vi "MTM2_getSample_tangentActuatorSteps.vi"(8 "error in (no error)":errorcluster, 11 "tangentActuatorSteps_Ctl":T1={"private_rcvStamp"=0.0, "steps[6]"=[0, 0, 0, 0, 0, 0]}) -> (0 "error out":errorcluster, 2 "function return":i32, 3 "tangentActuatorSteps_Ctl out":T1)   [LabVIEW 2018, in "SALLV_MTM2.lvlib"]
doc: "int MTM2_shm_getSample_tangentActuatorStepsLV(MTM2_tangentActuatorStepsLV *tangentActuatorSteps_Ctl );"
uses:
  DataTypes/tangentActuatorSteps.ctl
  SALLV_MTM2.lvlib
  SALLV_MTM2.so
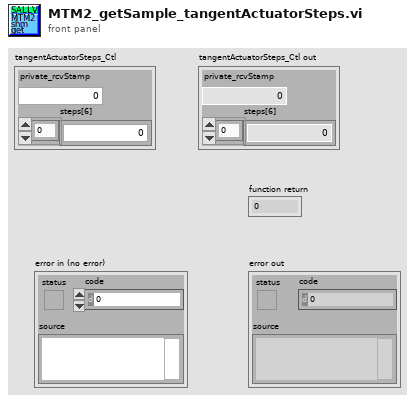
[diagram p1: front panel]
types:
  T1 = typedef "SALLV_MTM2.lvlib/tangentActuatorSteps.ctl" = cluster{"private_rcvStamp":dbl, "steps[6]":i32[]}
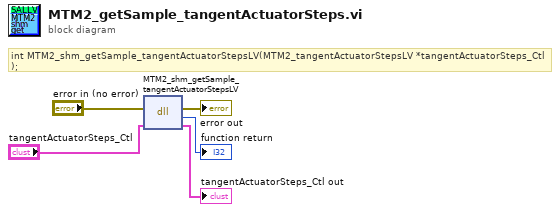
[diagram p0: block diagram]
diagram:
  # "int MTM2_shm_getSample_tangentActuatorStepsLV(MTM2_tangentActuatorStepsLV *tangentActuatorSteps_Ctl );"
  n1 = dll-call lib="home/ttsai/Documents/salLabviewApi/SALLV_MTM2/SALLV_MTM2.*" fn="MTM2_shm_getSample_tangentActuatorStepsLV"(error in="error in (no error)", "tangentActuatorSteps_Ctl"="tangentActuatorSteps_Ctl") -> (error out=→"error out":errorcluster, →"function return":i32, "tangentActuatorSteps_Ctl"=→"tangentActuatorSteps_Ctl out":T1)  [unwired: 2 in, 1 out]
